vi "Analog Input - N Channels - Continuous Sampling.vi"() -> ()   [LabVIEW 2019]
uses:
  <vilib>/myRIO/Instrument Drivers/Onboard IO/AI Continuous/typedefs/AI Continuous Reference.ctl
  <vilib>/myRIO/Common/Instrument Driver Framework/Utilities/typedefs/myRIO Generic Hardware Reference.ctl
  <vilib>/myRIO/Common/Instrument Driver Framework/Utilities/typedefs/Hardware Version Enum.ctl
  <vilib>/myRIO/Common/Instrument Driver Framework/Utilities/typedefs/myRIO v1.0 Reference.ctl
  <vilib>/myRIO/Common/Instrument Driver Framework/Utilities/typedefs/Generic FPGA Reference.ctl
  <vilib>/myRIO/Common/Instrument Driver Framework/ELVIS III v1.0/AI Continuous/typedefs/AI Continuous Channels List.ctl
  <vilib>/myRIO/Common/Instrument Driver Framework/ELVIS III v1.0/AI Continuous/typedefs/ELVIS III v1.0 AI Continuous Channels Enum.ctl
  <vilib>/myRIO/Common/Instrument Driver Framework/Utilities/typedefs/Analog Scaling Constants.ctl
  <vilib>/userdefined/High Color/nirio_resource_hc.ctl
  <vilib>/myRIO/Common/Instrument Driver Framework/ELVIS III v1.0/AI Continuous/vis/ELVIS III v1.1 Open AI (Continuous).vi
  <vilib>/myRIO/Common/Instrument Driver Framework/Utilities/vis/Validate Channels.vi
  <vilib>/myRIO/Common/Instrument Driver Framework/ELVIS III v1.0/AI Continuous/vis/ELVIS III v1.0 Reserve AI Continuous.vi
  <vilib>/myRIO/Common/Instrument Driver Framework/ELVIS III v1.0/AI Continuous/vis/ELVIS III v1.0 Close AI Continuous.vi
  <vilib>/myRIO/Common/Instrument Driver Framework/myRIO v1.0/UART/vis/myRIO v1.0 Close UART.vi
  <vilib>/myRIO/Common/Instrument Driver Framework/ELVIS III v1.0/AI Continuous/vis/ELVIS III v1.0 Build MUX Configuration AI Continuous.vi
  <vilib>/myRIO/Common/Instrument Driver Framework/ELVIS III v1.0/AI Continuous/vis/ELVIS III v1.0 Unreserve AI Continuous.vi
  <vilib>/Utility/VariantDataType/GetNumericInfo.vi
  <vilib>/Utility/error.llb/Error Cluster From Error Code.vi
  <vilib>/myRIO/Common/Instrument Driver Framework/ELVIS III v1.0/ELVIS III v1.1 Open.vi
  <vilib>/myRIO/Common/Instrument Driver Framework/ELVIS III v1.0/Resource Manager/vis/ELVIS III v1.0 Coerce AI Scaling.vi
  <vilib>/myRIO/Common/Instrument Driver Framework/ELVIS III v1.0/Resource Manager/vis/ELVIS III v1.0 Reserve Channel List.vi
  <vilib>/myRIO/Common/Instrument Driver Framework/ELVIS III v1.0/Resource Manager/vis/ELVIS III v1.0 Configure DMAs.vi
  <vilib>/myRIO/Common/Instrument Driver Framework/myRIO v1.0/myRIO v1.0 Close.vi
  <vilib>/myRIO/Common/Instrument Driver Framework/ELVIS III v1.0/AI Continuous/vis/ELVIS III v1.1 Stop AI Continuous.vi
  <vilib>/myRIO/Common/Instrument Driver Framework/ELVIS III v1.0/AI Continuous/vis/ELVIS III v1.1 Start AI Continuous.vi
  <vilib>/myRIO/Common/Instrument Driver Framework/ELVIS III v1.0/AI Continuous/vis/ELVIS III v1.0 AI Continuous Read.vi
  <vilib>/myRIO/Common/Instrument Driver Framework/ELVIS III v1.0/Resource Manager/vis/ELVIS III v1.0 Unreserve Channel List.vi
  <vilib>/myRIO/Common/Instrument Driver Framework/Utilities/vis/FPGA Ref Manager.vi
  <vilib>/myRIO/Common/Instrument Driver Framework/ELVIS III v1.0/ELVIS III v1.0 Reset FPGA.vi
  <vilib>/myRIO/Common/Instrument Driver Framework/myRIO v1.0/IRQ/vis/myRIO v1.0 IRQ Info FGV.vi
  <vilib>/myRIO/Common/Instrument Driver Framework/myRIO v1.0/IRQ/vis/myRIO v1.0 Timer IRQ Info FGV.vi
  <vilib>/myRIO/Common/Instrument Driver Framework/myRIO v1.0/IRQ/vis/myRIO v1.0 ISR Agent.vi
  <vilib>/myRIO/Instrument Drivers/Utilities/vis/Reset Index.vi
  <vilib>/myRIO/Common/Instrument Driver Framework/myRIO v1.0/Resource Manager/vis/myRIO v1.0 Block Write Resource Manager.vi
  <vilib>/myRIO/Instrument Drivers/Onboard IO/AI Continuous/vis/myRIO AI Continuous Open.xnode
  <vilib>/myRIO/Instrument Drivers/Utilities/Utilities.lvlib
  <vilib>/myRIO/Instrument Drivers/Onboard IO/AI Continuous/AI Continuous.lvlib
panel:
  in  "Stop":bool
  in  "Acquire Data":bool
  out "Analog Data":dbl[][](graph)
  # "ELVIS III Control IO"
  # "模拟输入N通道"
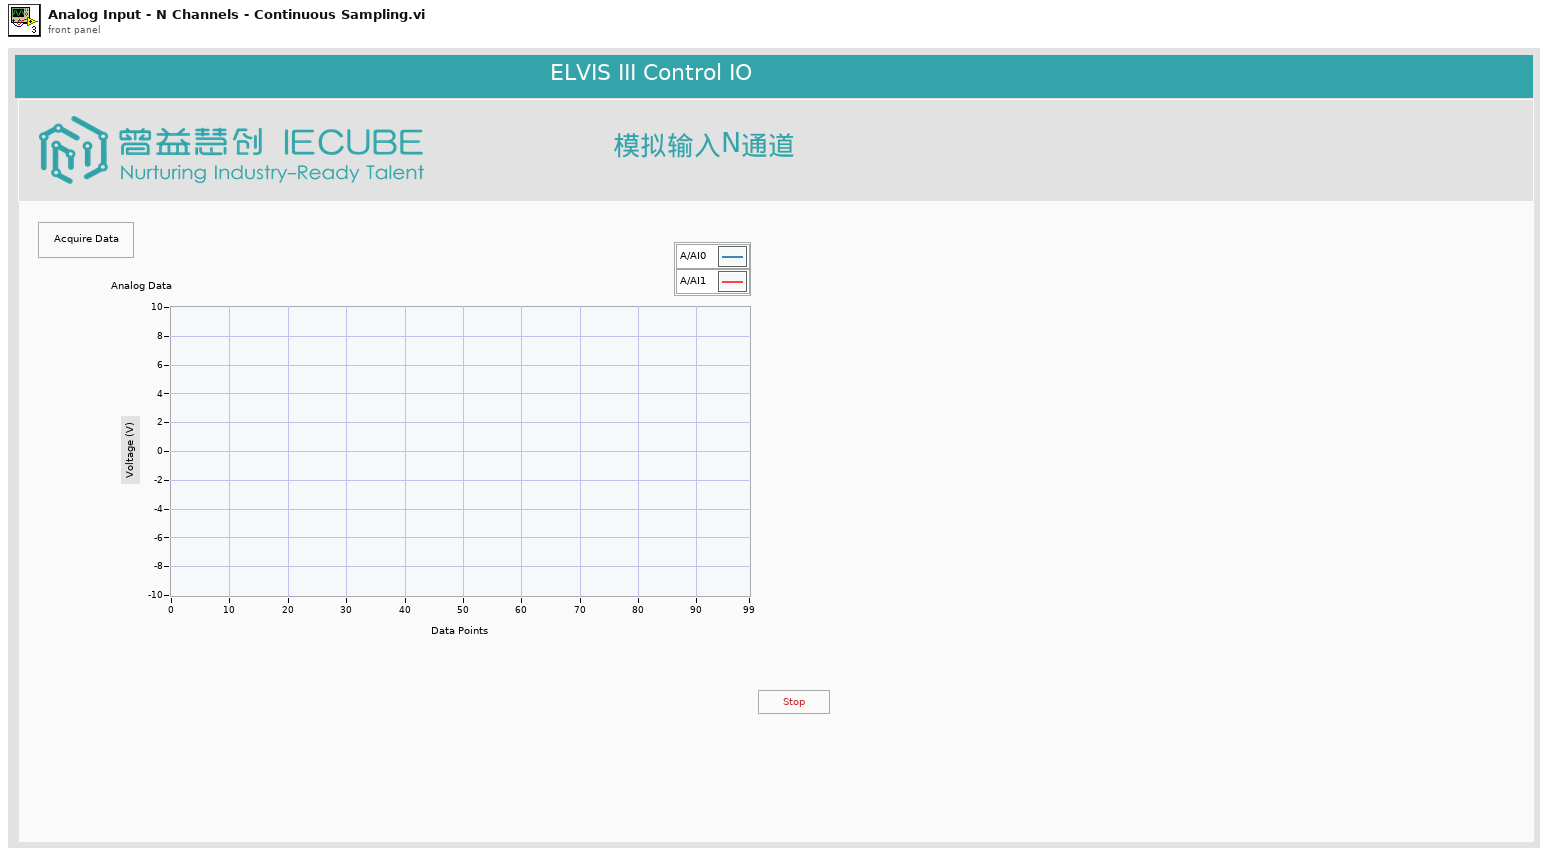
[diagram p1: front panel]
types:
  T1 = typedef "nirio_resource_hc.ctl" = tag
  T2 = typedef "Hardware Version Enum.ctl" = enum16{"Unknown", "myRIO-1900", "myRIO-1950", "roboRIO", "NI ELVIS RIO CM", "ELVIS III"}
  T3 = typedef "AI Continuous.lvlib/AI Continuous Reference.ctl" = cluster{"myRIO Reference":T4, "AI (Continuous) Channels List":T7, "AI (Continuous) Scaling Constants List":T9[], "Bank Count":u8[]}
  T4 = typedef "myRIO Generic Hardware Reference.ctl" = cluster{"myRIO Model":T2, "myRIO Hardware Reference":T5}
  T5 = typedef "myRIO v1.0 Reference.ctl" = cluster{"Generic FPGA Reference":T6, "Allow multiple opens":bool}
  T6 = typedef "Generic FPGA Reference.ctl" = refnum<k20>
  T7 = typedef "AI Continuous Channels List.ctl" = T8[]
  T8 = typedef "ELVIS III v1.0 AI Continuous Channels Enum.ctl" = enum16{"Not Connected", "A/AI0 (Continuous)", "A/AI1 (Continuous)", "A/AI2 (Continuous)", "A/AI3 (Continuous)", "A/AI4 (Continuous)", "A/AI5 (Continuous)", "A/AI6 (Continuous)", "A/AI7 (Continuous)", "A/AI0 (DIFF Continuous)", "A/AI1 (DIFF Continuous)", "A/AI2 (DIFF Continuous)", "A/AI3 (DIFF Continuous)", "B/AI0 (Continuous)", "B/AI1 (Continuous)", "B/AI2 (Continuous)", "B/AI3 (Continuous)", "B/AI4 (Continuous)", "B/AI5 (Continuous)", "B/AI6 (Continuous)", "B/AI7 (Continuous)", "B/AI0 (DIFF Continuous)", "B/AI1 (DIFF Continuous)", "B/AI2 (DIFF Continuous)", "B/AI3 (DIFF Continuous)"}
  T9 = typedef "Analog Scaling Constants.ctl" = cluster{"LSB Weight (Volts)":dbl, "Offset (Volts)":dbl, "Signed?":bool}
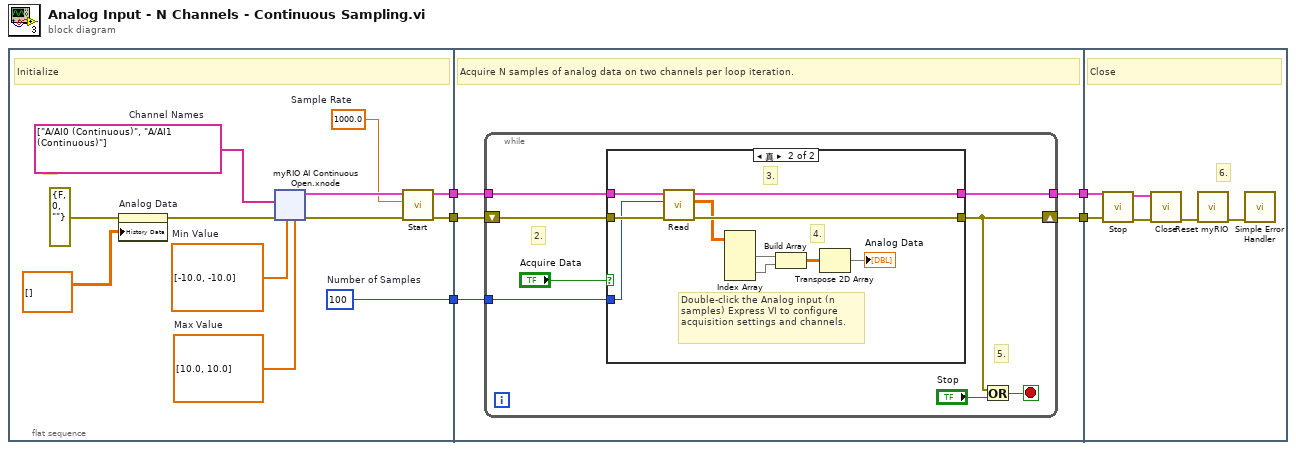
[diagram p0: block diagram]
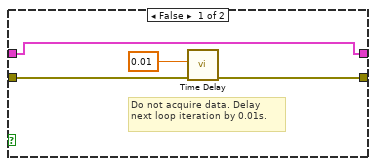
[diagram p2: hidden frame]
diagram:
  n1 = flat-sequence {
    tunnel: [w13] -> w5
    tunnel: [w14] -> w4
    tunnel: [w15] -> w3
    tunnel: [w43] -> w2
    tunnel: w5 -> [w42]
    tunnel: w4 -> [w41]
    tunnel: w3 -> [w40]
    tunnel: [w39] -> w1
    tunnel: w2 -> [w70]
    tunnel: w1 -> [w67]
    frame #0 {
      w6 = 1000.0  # Sample Rate
      w10 = tag[] ["A/AI0 (Continuous)", "A/AI1 (Continuous)"]  # Channel Names
      w15 = u32 100  # Number of Samples
      w9 = dbl[] [10.0, 10.0]  # Max Value
      w8 = dbl[] [-10.0, -10.0]  # Min Value
      # "1."
      # "Initialize"
      n2 = property on="Analog Data" class="WFChart (严格)"(error in=errorcluster {"status"=FALSE, "code"=0, "source"=""} ("error in (no error)"), "History Data"=dbl[][] []) -> (error out=w11:errorcluster)  [unwired: 1 in, 1 out]
      n3 = xnode "myRIO AI Continuous Open.xnode"("error in (no error)"=w11, "Channel Names"=w10, "Max Value"=w9, "Min Value"=w8) -> ("error out"=w12:errorcluster, "AI (Continuous) Ref Out"=w7:T3)
      n4 = call <vilib>:"Start.vi"("error in (no error)"=w12, "Sample Rate"=w6, "AI (Continuous) Ref In"=w7) -> ("error out"=w13:errorcluster, "AI (Continuous) Ref Out"=w14:T3)  [unwired: 7 in]
    }
    frame #1 {
      # "Acquire N samples of analog data on two channels per loop iteration."
      n5 = while {
        shift-right: [w49] -> w43
        shift-left: w42 -> [w50]
        tunnel: w41 -> [w44]
        tunnel: w40 -> [w46]
        tunnel: [w45] -> w39
        stop <- w51 stop-if-true
        # "5."
        # "2."
        n6 = case shown="真" "Acquire Data" {
          tunnel: w50 -> [w54 w61]
          tunnel: [w53 w60] -> w49
          tunnel: w46 -> [_ w57]
          tunnel: [w52 w58] -> w45
          tunnel: w44 -> [w52 w56]
          frame False {
            # "Do not acquire data. Delay next loop iteration by 0.01s."
            n7 = call "Time Delay"("error in (no error)"=w54, "Delay Time (s)"=0.01) -> ("error out"=w53:errorcluster)  [unwired: 9 in]
          }
          frame True {
            # "4."
            # "3."
            # "Double-click the Analog input (n samples) Express VI to configure acquisition settings and channels."
            n8 = call <vilib>:"Read.vi"("error in (no error)"=w61, "Number of Samples"=w57, "AI (Continuous) Ref In"=w56) -> ("error out"=w60:errorcluster, "Values"=w59:dbl[][], "AI (Continuous) Ref Out"=w58:T3)  [unwired: 6 in]
            n9 = Index Array(array=w59) -> (element #1=w65:dbl[], element #2=w64:dbl[])  [unwired: 4 in]
            n10 = Build Array(w65, w64) -> (w63:dbl[][])
            n11 = Transpose 2D Array(2D array=w63) -> (transposed array=→"Analog Data":dbl[][])
          }
        }
        n12 = Or(x=w49, y="Stop") -> (x .or. y?=w51:bool)
      }
    }
    frame #2 {
      # "6."
      # "Close"
      n13 = call <vilib>:"Stop.vi"("error in (no error)"=w70, "AI (Continuous) Ref In"=w67) -> ("error out"=w69:errorcluster, "AI (Continuous) Ref Out"=w66:T3)  [unwired: 8 in]
      n14 = call <vilib>:"Close.vi"("error in (no error)"=w69, "AI (Continuous) Ref In"=w66) -> ("error out"=w68:errorcluster)  [unwired: 9 in]
      n15 = call <vilib>:"Reset myRIO.vi"("error in (no error)"=w68) -> ("error out"=w71:errorcluster)  [unwired: 10 in]
      n16 = call <vilib>:"Simple Error Handler.vi"("error in (no error)"=w71) -> ()  [unwired: 4 in, 5 out]
    }
  }
